vi "im going insane.vi"(8 "control frequency calculated":dbl=20.0, 9 "Distance":dbl, 10 "Velocity Max":dbl=10.0, 11 "Acceleration Max":dbl=30.0) -> (2 "Velocity values":dbl[](array[numeric]), 3 "Timestamp":dbl[](array[numeric]) format="%.2f")   [LabVIEW 2020]
panel:
  out "Time":sgl
  out "XY Graph":cluster{dbl[], dbl[]}(graph)
  out "Time(othy) (in seconds)":dbl
  # "*timeothy is the point where the slope changes in a trapezoid"
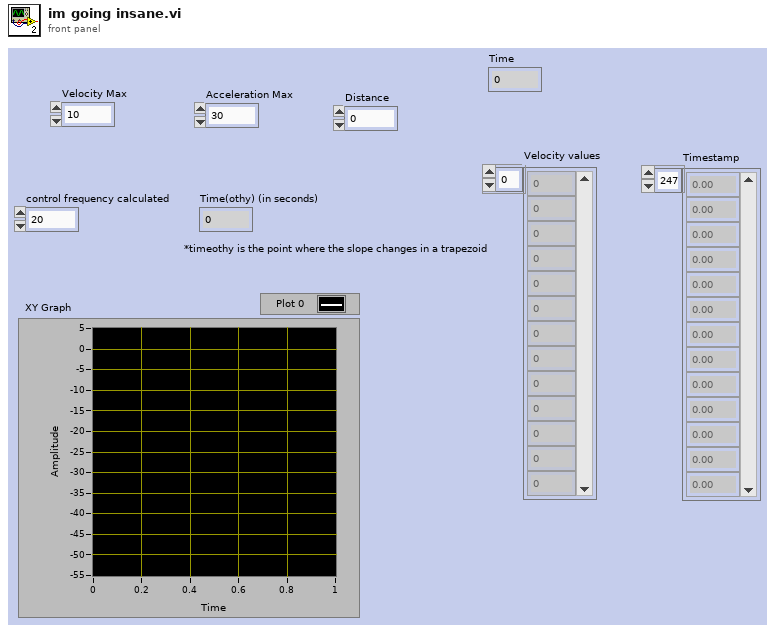
[diagram p1: front panel]
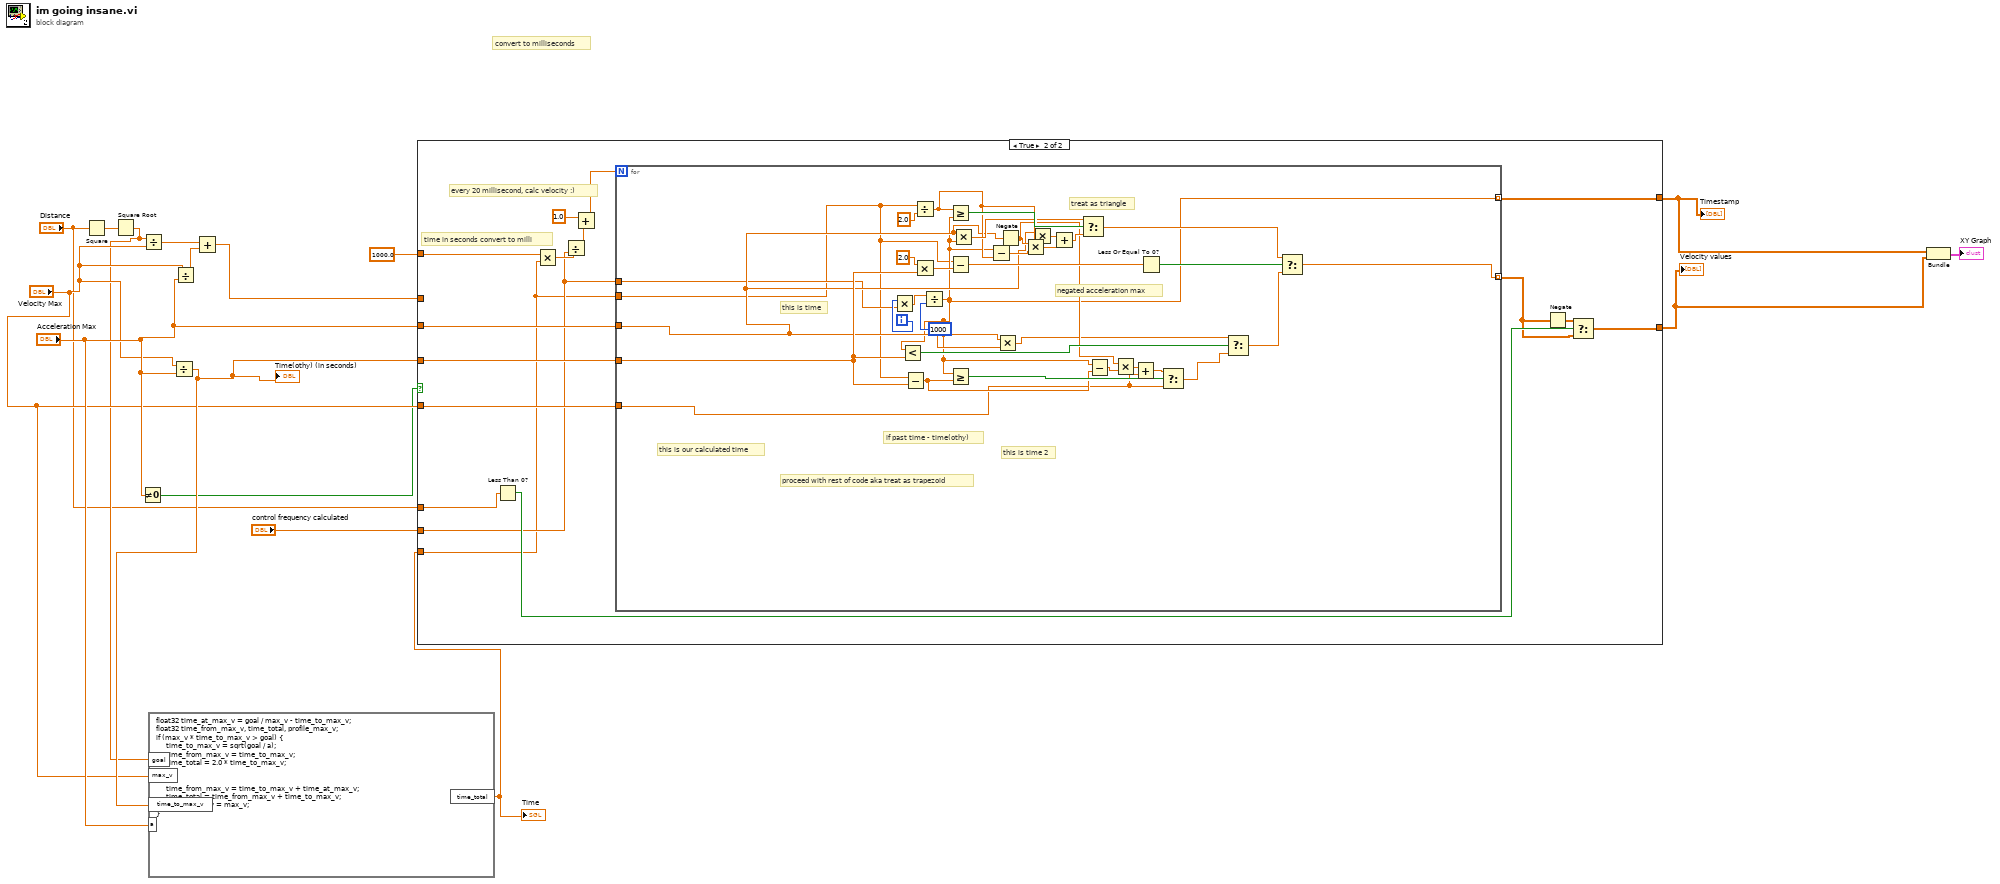
[diagram p0: block diagram]
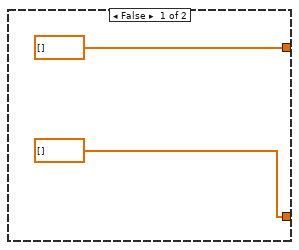
[diagram p2: hidden frame]
diagram:
  # "convert to milliseconds"
  n1 = Square(x="Distance") -> (x^2=w3:dbl)
  n2 = Square Root(x=w3) -> (sqrt(x)=w2:dbl)
  n3 = Not Equal To 0?(x="Acceleration Max") -> (x != 0?=w4:bool)
  n4 = Divide(x=w2, y="Velocity Max") -> (x/y=w12:dbl)
  n5 = Divide(x="Velocity Max", y="Acceleration Max") -> (x/y=w6:dbl)
  "Time(othy) (in seconds)" <- w6
  n6 = formula code="float32 time_at_max_v = goal / max_v - time_to_max_v;\nfloat32 time_from_max_v, time_total, profile_max_v;\nif (max_v * time_to_max_v > goal) {\n     time_to_max_v = sqrt(goal / a);\n     time_from_max_v = time_to_max_v;\n     time_total = 2.0 * time_to_max_v;\n}\nelse {\n     time_from_max_v = time_to_max_v + time_at_max_v;\n     time_total = time_from_max_v + time_to_max_v;\n     profile_max_v = max_v;\n}"("goal"=w2, "max_v"="Velocity Max", "time_to_max_v"=w6, "a"="Acceleration Max") -> ("time_total"=w8:sgl)
  "Time" <- w8
  n7 = Divide(x="Velocity Max", y="Acceleration Max") -> (x/y=w16:dbl)
  n8 = Add(x=w12, y=w16) -> (x+y=w13:dbl)
  n9 = case shown="True" w4 {
    tunnel: "Velocity Max" -> [_ w34]
    tunnel: w6 -> [_ w33]
    tunnel: 1000.0 ("x") -> [_ w32]
    tunnel: [dbl[] [] w30] -> w14
    tunnel: w13 -> [_ _]
    tunnel: "Acceleration Max" -> [_ w26]
    tunnel: [dbl[] [] w22] -> w11
    tunnel: "control frequency calculated" -> [_ w21]
    tunnel: w8 -> [_ w19]
    tunnel: "Distance" -> [_ w20]
    frame False {
    }
    frame True {
      # "every 20 millisecond, calc velocity :)"
      # "time in seconds convert to milli"
      n10 = Less Than 0?(x=w20) -> (x < 0?=w24:bool)
      n11 = Multiply(x=w32, y=w19) -> (x*y=w31:dbl)
      n12 = Divide(x=w31, y=w21) -> (x/y=w27:dbl)
      n13 = Add(x=1.0, y=w27) -> (x+y=w29:dbl)
      n14 = for {
        N: w29 -> [_]
        tunnel: [w57] -> w23 mode=indexing
        tunnel: w26 -> [w47]
        tunnel: w34 -> [w39]
        tunnel: w33 -> [w56]
        tunnel: [w37] -> w30 mode=indexing
        tunnel: w21 -> [w36]
        tunnel: w19 -> [w35]
        i -> [w38]
        # "this is our calculated time"
        # "this is time 2"
        # "this is time"
        # "negated acceleration max"
        # "if past time - time(othy)"
        # "treat as triangle"
        # "proceed with rest of code aka treat as trapezoid"
        n15 = Multiply(x=w38, y=w36) -> (x*y=w44:dbl)
        n16 = Subtract(x=w35, y=w56) -> (x-y=w45:dbl)
        n17 = Divide(x=w35, y=2.0) -> (x/y=w50:dbl)
        n18 = Multiply(x=2.0, y=w56) -> (x*y=w66:dbl)
        n19 = Divide(x=w44, y=1000) -> (x/y=w37:dbl)
        n20 = Less?(x=w37, y=w56) -> (x < y?=w58:bool)
        n21 = Greater Or Equal?(x=w50, y=w37) -> (x >= y?=w62:bool)
        n22 = Subtract(x=w35, y=w66) -> (x-y=w65:dbl)
        n23 = Greater Or Equal?(x=w37, y=w45) -> (x >= y?=w61:bool)
        n24 = Multiply(x=w47, y=w37) -> (x*y=w55:dbl)
        n25 = Subtract(x=w37, y=w50) -> (x-y=w54:dbl)
        n26 = Multiply(x=w37, y=w47) -> (x*y=w42:dbl)
        n27 = Negate(x=w47) -> (-x=w49:dbl)
        n28 = Multiply(x=w49, y=w54) -> (x*y=w53:dbl)
        n29 = Multiply(x=w47, y=w50) -> (x*y=w52:dbl)
        n30 = Add(x=w52, y=w53) -> (x+y=w51:dbl)
        n31 = Select(t=w55, s=w62, f=w51) -> (s? t:f=w46:dbl)
        n32 = Subtract(x=w37, y=w45) -> (x-y=w40:dbl)
        n33 = Multiply(x=w49, y=w40) -> (x*y=w48:dbl)
        n34 = Add(x=w48, y=w39) -> (x+y=w41:dbl)
        n35 = Less Or Equal To 0?(x=w65) -> (x <= 0?=w64:bool)
        n36 = Select(t=w41, s=w61, f=w39) -> (s? t:f=w60:dbl)
        n37 = Select(t=w42, s=w58, f=w60) -> (s? t:f=w59:dbl)
        n38 = Select(t=w46, s=w64, f=w59) -> (s? t:f=w57:dbl)
      }
      n39 = Negate(x=w23) -> (-x=w25:dbl[])
      n40 = Select(t=w25, s=w24, f=w23) -> (s? t:f=w22:dbl[])
    }
  }
  "Velocity values" <- w11
  "Timestamp" <- w14
  n41 = Bundle(w14, w11) -> (→"XY Graph":cluster{dbl[], dbl[]})  [unwired: 1 in]
